vi "测量流程.vi"(11 "控制命令":T1(ring)) -> ()   [LabVIEW 2016, in "斯坦道总磷总氮.lvlib"]
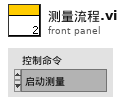
[diagram p1: front panel]
types:
  T1 = enum16{"启动测量", "标样核查", "零点核查", "跨度核查", "空白测试", "平行样测试", "加标回收", "空白校准", "标样校准", "初始化（清洗）", "停止测试", "仪器重启", "校时", "模式设置", "测量间隔设置"}
  T2 = typedef "斯坦道总磷总氮.lvlib/测试流程控件.ctl" = enum16{"初始化", "参数1启动", "参数1测试中", "参数1测试结束", "参数2启动", "参数2测试中", "参数2测试结束", "参数3启动", "参数3测试中", "参数3测试结束", "流程结束"}
  T3 = cluster{"时间标识":timestamp, "设备":string, "日志信息":string, "流程参数":string}
  T4 = cluster{"站号":u16, "量程切换":enum32{"H", "L", "AUTO"}, "控制命令":enum16{"启动测量", "标样核查", "零点核查", "跨度核查", "空白测试", "平行样测试", "加标回收", "空白校准", "标样校准", "初始化（清洗）", "停止测试", "仪器重启", "校时", "模式设置", "测量间隔设置"}, "模式设置":enum16{"待机", "连续模式", "周期模式", "定点模式", "受控模式", "手动模式"}, "测量间隔":u16}
  T5 = enum16{"空闲", "水样测试", "标样核查", "零点核查", "跨度核查", "空白测试", "平行样测试", "加标回收", "空白校准", "标样校准", "初始化（清洗）"}
  T6 = cluster{"系统时间":timestamp, "工作状态":enum16{"空闲", "水样测试", "标样核查", "零点核查", "跨度核查", "空白测试", "平行样测试", "加标回收", "空白校准", "标样校准", "初始化（清洗）"}, "测量模式":enum16{"待机", "连续模式", "周期模式", "定点模式", "受控模式", "手动模式"}, "告警代码":enum16{"无告警", "缺试剂告警", "缺水样告警", "缺蒸馏水告警", "缺标液告警", "仪表漏液告警", "标定异常告警", "超量程告警", "加热异常", "低试剂预警", "超上限告警", "超下限告警", "仪表内部其他异常", "滴定异常告警", "电极异常告警", "量程切换告警", "参数设置告警", "PH电极电位异常", "电导率电极异常", "浊度光度异常", "溶解氧电极异常", "溶解氧光强异常", "温度异常告警", "PH异常告警", "溶解氧异常告警", "电导率异常告警", "浊度异常告警", "叶绿素异常告警", "藻密度异常告警", "蓝绿藻异常告警", "ORP异常告警", "氨氮异常告警", "清洁刷异常告警", "SD卡异常告警", "蓝牙异常告警", "Wifi异常告警", "流程异常告警"}, "故障代码":enum16{"无故障", "电机故障", "温度故障", "通讯故障", "滴定故障"}, "日志代码":u16, "软件版本":u16, "F0":sgl, "F1":sgl, "F2":sgl, "F3":sgl, "T":sgl, "H":sgl, "id":u16, "flowid":u16, "量程":u16, "总磷控温温度1":sgl, "营养盐控温温度2":sgl, "ADC":sgl}
  T7 = cluster{"水样测试量程模式":enum16{"H", "L", "AUTO"}, "空白核查量程模式":enum16{"H", "L", "AUTO"}, "跨度核查量程模式":enum16{"H", "L", "AUTO"}}
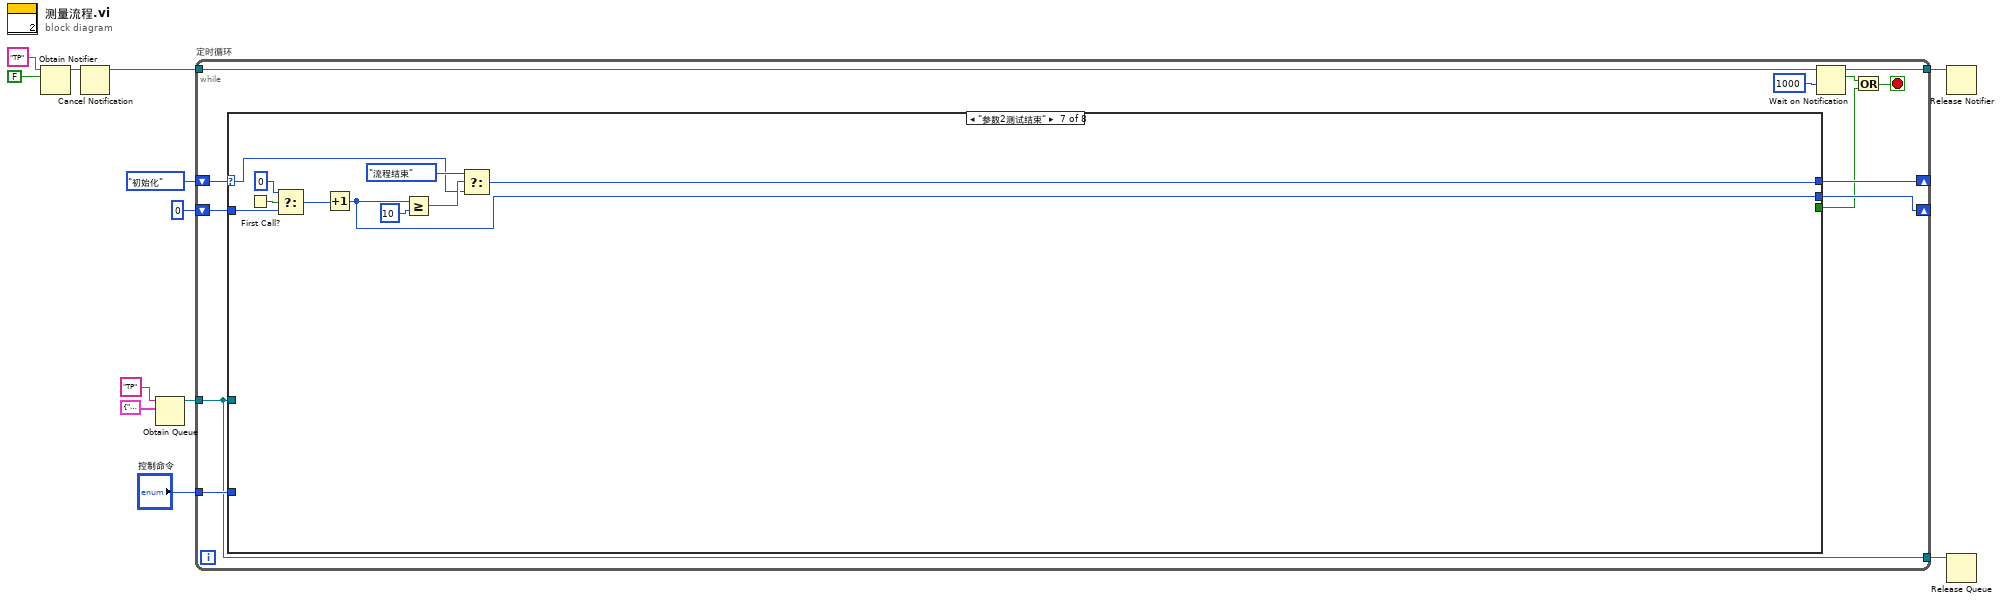
[diagram p0: block diagram]
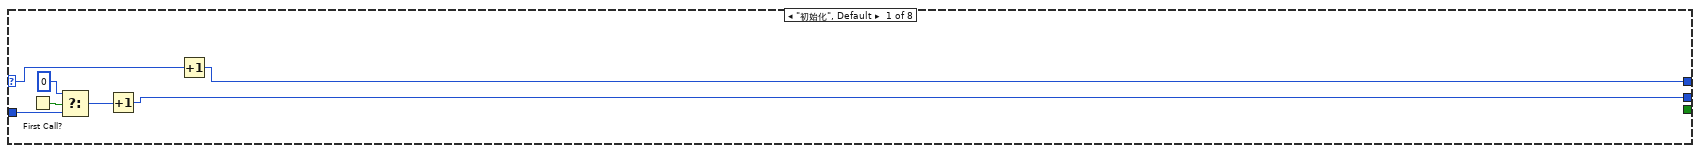
[diagram p2: hidden frame]
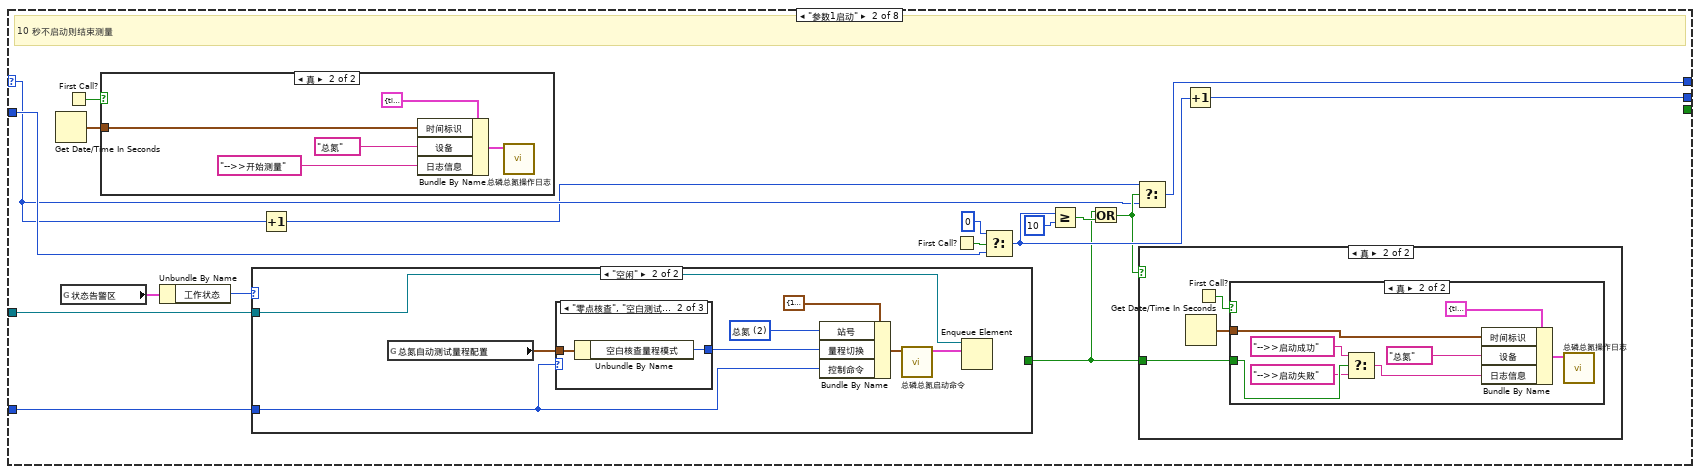
[diagram p3: hidden frame]
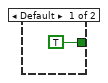
[diagram p7: hidden frame]
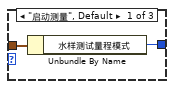
[diagram p8: hidden frame]
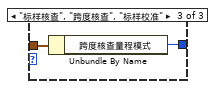
[diagram p9: hidden frame]
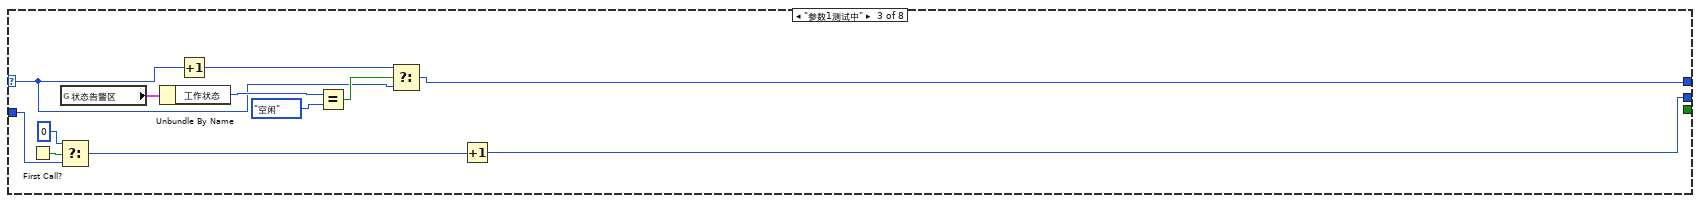
[diagram p10: hidden frame]
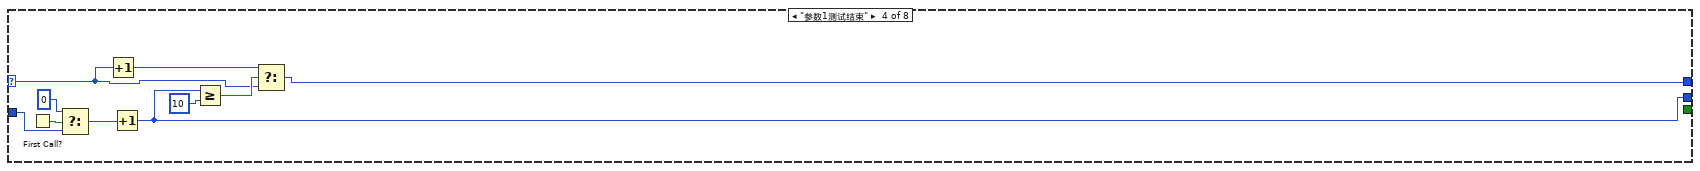
[diagram p11: hidden frame]
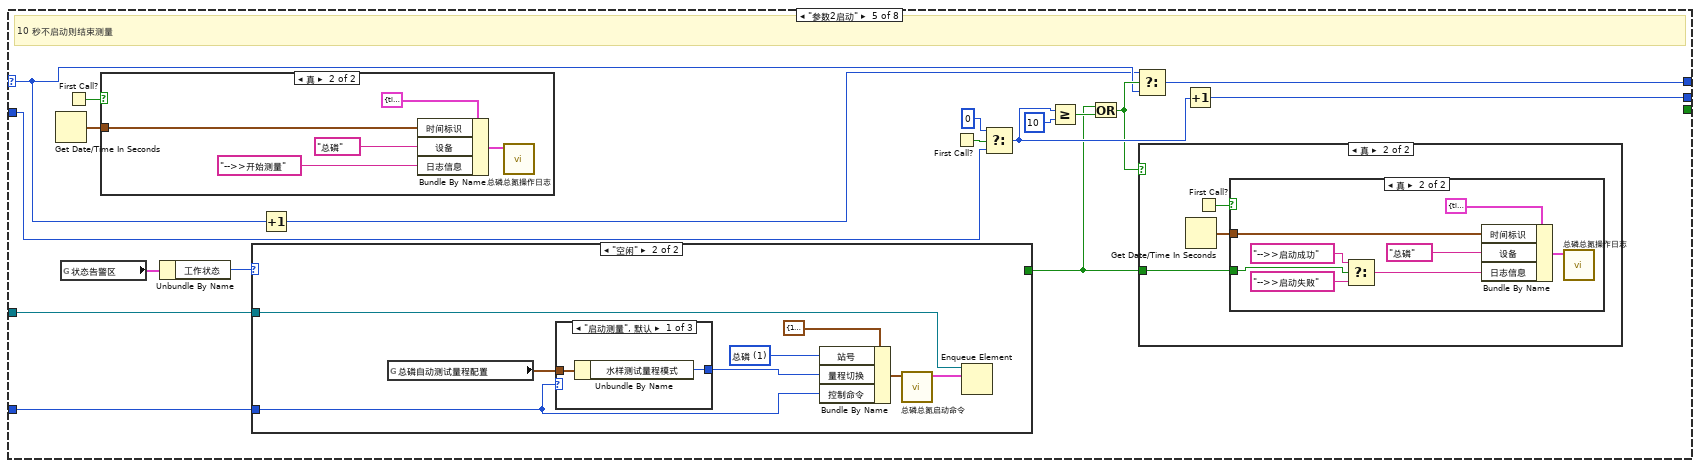
[diagram p12: hidden frame]
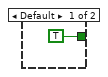
[diagram p16: hidden frame]
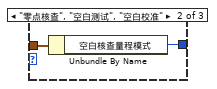
[diagram p17: hidden frame]
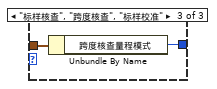
[diagram p18: hidden frame]
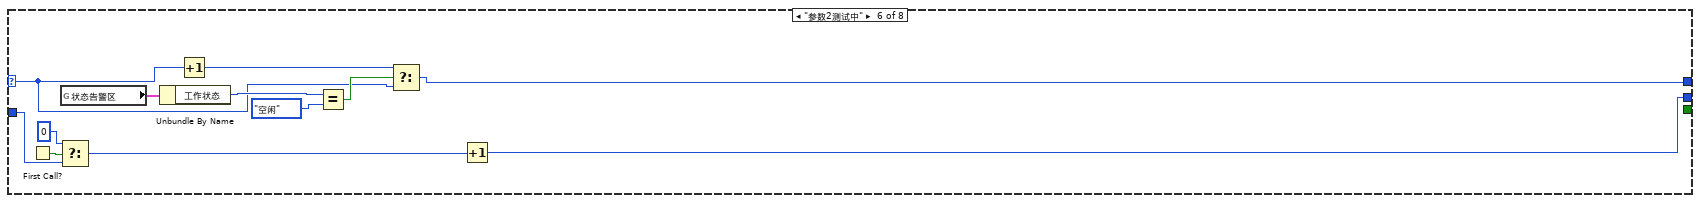
[diagram p19: hidden frame]
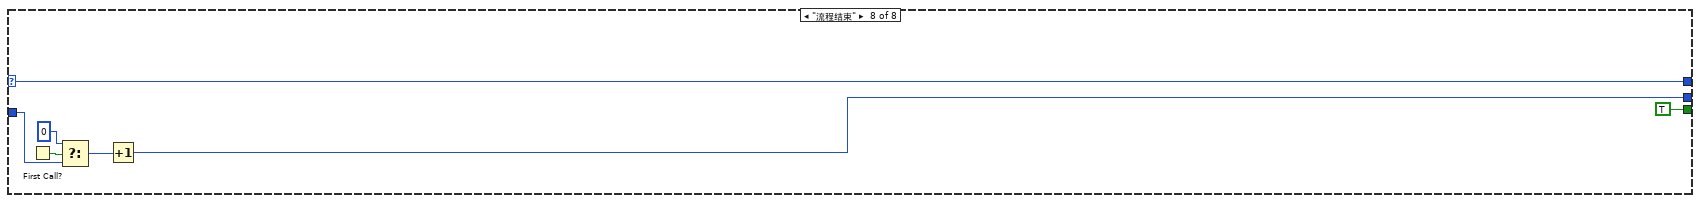
[diagram p20: hidden frame]
diagram:
  n1 = Obtain Notifier(name (unnamed)="TP" ("名称（未命名）"), notification data type=FALSE) -> (notifier out=w7:refnum<notifier>)  [unwired: 2 in, 2 out]
  n2 = Cancel Notification(0:w7) -> (8:w6:refnum<notifier>)  [unwired: 1 in, 2 out]
  n3 = Obtain Queue(name (unnamed)="TP" ("名称（未命名）"), element data type=cluster{"命令":string, "data":variant} {"命令"="", "data"=variant}) -> (queue out=w10:refnum<queue>)  [unwired: 3 in, 2 out]
  n4 = while "定时循环" {
    tunnel: w10 -> [w13]
    tunnel: w6 -> [w24]
    tunnel: "控制命令" -> [w19]
    shift-right: [w18] -> _
    shift-left: 测试流程控件."初始化" -> [w20]
    shift-right: [w16] -> _
    shift-left: 0 -> [w17]
    tunnel: [w14] -> w2
    tunnel: [w13] -> w3
    stop <- w21 stop-if-true
    n5 = case shown="\"参数2测试结束\"" w20 {
      selector: w20 -> [w31 w35 w83 w94 w106 w154 w165 w179]
      tunnel: w19 -> [_ w49 _ _ w120 _ _ _]
      tunnel: w13 -> [_ w48 _ _ w119 _ _ _]
      tunnel: [w30 w39 w84 w93 w110 w155 w164 w179] -> w18
      tunnel: w17 -> [w28 w43 w90 w100 w114 w161 w171 w175]
      tunnel: [w25 w42 w81 w98 w113 w152 w169 w174] -> w16
      tunnel: [_ _ _ _ _ _ _ TRUE] -> w15
      frame "初始化", Default {
        n6 = First Call?() -> (First Call?: T/F=w29:bool)
        n7 = Select(t=0, s=w29, f=w28) -> (s? t:f=w26:i32)
        n8 = Increment(x=w26) -> (x+1=w25:i32)
        n9 = Increment(x=w31) -> (x+1=w30:T2)
      }
      frame "参数1启动" {
        # "10 秒不启动则结束测量"
        n10 = Get Date/Time In Seconds() -> (seconds since 1Jan1904=w33:timestamp)
        n11 = global read "VAR总磷总氮全局变量.vi" "状态告警区"() -> (w47:T6)
        n12 = First Call?() -> (First Call?: T/F=w32:bool)
        n13 = case shown="真" w32 {
          tunnel: w33 -> [_ w53]
          frame False {
          }
          frame True {
            n14 = Bundle By Name(cluster=T3 {"时间标识"=timestamp(0 s since 1904-01-01), "设备"="", "日志信息"="", "流程参数"=""} ("data in"), "时间标识"=w53, "设备"="总氮" ("组合框"), "日志信息"="-->>开始测量") -> (w54:T3)
            n15 = call "总磷总氮操作日志.vi"("data in"=w54) -> ()  [unwired: 11 in]
          }
        }
        n16 = Unbundle By Name(w47) -> ("工作状态"=w46:T5)
        n17 = case shown="\"空闲\"" w46 {
          tunnel: w49 -> [_ w68]
          tunnel: w48 -> [_ w72]
          tunnel: [TRUE _] -> w36
          frame Default {
          }
          frame "空闲" {
            w71 = u16 2 items=["总磷"=1, "总氮"=2, "氨氮"=3, "COD"=22] ("站号")
            n18 = global read "总磷总氮断电保存全局变量.vi" "总氮自动测试量程配置"() -> (w67:T7)
            n19 = case shown="\"零点核查\", \"空白测试\", \"空白校准\"" w68 {
              tunnel: w67 -> [w76 w78 w80]
              tunnel: [w75 w77 w79] -> w74
              frame "启动测量", Default {
                n20 = Unbundle By Name(w76) -> ("水样测试量程模式"=w75:enum16{"H", "L", "AUTO"})
              }
              frame "零点核查", "空白测试", "空白校准" {
                n21 = Unbundle By Name(w78) -> ("空白核查量程模式"=w77:enum16{"H", "L", "AUTO"})
              }
              frame "标样核查", "跨度核查", "标样校准" {
                n22 = Unbundle By Name(w80) -> ("跨度核查量程模式"=w79:enum16{"H", "L", "AUTO"})
              }
            }
            n23 = Bundle By Name(cluster=T4 {"站号"=1, "量程切换"=enum."AUTO", "控制命令"=enum."启动测量", "模式设置"=enum."待机", "测量间隔"=0} ("参数"), "站号"=w71, "量程切换"=w74, "控制命令"=w68) -> (w69:T4)
            n24 = call "总磷总氮启动命令.vi"("参数"=w69) -> ("启动命令"=w73:cluster{"命令":string, "data":variant})  [unwired: 10 in]
            n25 = Enqueue Element(queue=w72, element=w73) -> ()  [unwired: 2 in, 3 out]
          }
        }
        n26 = Increment(x=w35) -> (x+1=w34:T2)
        n27 = First Call?() -> (First Call?: T/F=w45:bool)
        n28 = Select(t=0, s=w45, f=w43) -> (s? t:f=w41:i32)
        n29 = Greater Or Equal?(x=w41, y=10) -> (x >= y?=w38:bool)
        n30 = Or(x=w36, y=w38) -> (x .or. y?=w37:bool)
        n31 = Select(t=w34, s=w37, f=w35) -> (s? t:f=w39:T2)
        n32 = case shown="真" w37 {
          tunnel: w36 -> [_ w55]
          frame False {
          }
          frame True {
            n33 = Get Date/Time In Seconds() -> (seconds since 1Jan1904=w56:timestamp)
            n34 = First Call?() -> (First Call?: T/F=w57:bool)
            n35 = case shown="真" w57 {
              tunnel: w56 -> [_ w64]
              tunnel: w55 -> [_ w62]
              frame False {
              }
              frame True {
                n36 = Select(t="-->>启动成功" ("日志信息"), s=w62, f="-->>启动失败" ("日志信息")) -> (s? t:f=w59:string)
                n37 = Bundle By Name(cluster=T3 {"时间标识"=timestamp(0 s since 1904-01-01), "设备"="", "日志信息"="", "流程参数"=""} ("data in"), "时间标识"=w64, "设备"="总氮" ("组合框"), "日志信息"=w59) -> (w65:T3)
                n38 = call "总磷总氮操作日志.vi"("data in"=w65) -> ()  [unwired: 11 in]
              }
            }
          }
        }
        n39 = Increment(x=w41) -> (x+1=w42:i32)
      }
      frame "参数1测试中" {
        n40 = First Call?() -> (First Call?: T/F=w92:bool)
        n41 = Select(t=0, s=w92, f=w90) -> (s? t:f=w89:i32)
        n42 = global read "VAR总磷总氮全局变量.vi" "状态告警区"() -> (w88:T6)
        n43 = Unbundle By Name(w88) -> ("工作状态"=w87:T5)
        n44 = Increment(x=w83) -> (x+1=w82:T2)
        n45 = Equal?(x=w87, y=T5."空闲") -> (x = y?=w85:bool)
        n46 = Select(t=w82, s=w85, f=w83) -> (s? t:f=w84:T2)
        n47 = Increment(x=w89) -> (x+1=w81:i32)
      }
      frame "参数1测试结束" {
        n48 = First Call?() -> (First Call?: T/F=w102:bool)
        n49 = Select(t=0, s=w102, f=w100) -> (s? t:f=w99:i32)
        n50 = Increment(x=w94) -> (x+1=w95:T2)
        n51 = Increment(x=w99) -> (x+1=w98:i32)
        n52 = Greater Or Equal?(x=w98, y=10) -> (x >= y?=w96:bool)
        n53 = Select(t=w95, s=w96, f=w94) -> (s? t:f=w93:T2)
      }
      frame "参数2启动" {
        # "10 秒不启动则结束测量"
        n54 = Get Date/Time In Seconds() -> (seconds since 1Jan1904=w104:timestamp)
        n55 = global read "VAR总磷总氮全局变量.vi" "状态告警区"() -> (w118:T6)
        n56 = First Call?() -> (First Call?: T/F=w103:bool)
        n57 = case shown="真" w103 {
          tunnel: w104 -> [_ w124]
          frame False {
          }
          frame True {
            n58 = Bundle By Name(cluster=T3 {"时间标识"=timestamp(0 s since 1904-01-01), "设备"="", "日志信息"="", "流程参数"=""} ("data in"), "时间标识"=w124, "设备"="总磷" ("组合框"), "日志信息"="-->>开始测量") -> (w125:T3)
            n59 = call "总磷总氮操作日志.vi"("data in"=w125) -> ()  [unwired: 11 in]
          }
        }
        n60 = Unbundle By Name(w118) -> ("工作状态"=w117:T5)
        n61 = case shown="\"空闲\"" w117 {
          tunnel: w120 -> [_ w139]
          tunnel: w119 -> [_ w143]
          tunnel: [TRUE _] -> w107
          frame Default {
          }
          frame "空闲" {
            w142 = u16 1 items=["总磷"=1, "总氮"=2, "氨氮"=3, "COD"=22] ("站号")
            n62 = global read "总磷总氮断电保存全局变量.vi" "总磷自动测试量程配置"() -> (w138:T7)
            n63 = case shown="\"启动测量\", 默认" w139 {
              tunnel: w138 -> [w147 w149 w151]
              tunnel: [w146 w148 w150] -> w145
              frame "启动测量", Default {
                n64 = Unbundle By Name(w147) -> ("水样测试量程模式"=w146:enum16{"H", "L", "AUTO"})
              }
              frame "零点核查", "空白测试", "空白校准" {
                n65 = Unbundle By Name(w149) -> ("空白核查量程模式"=w148:enum16{"H", "L", "AUTO"})
              }
              frame "标样核查", "跨度核查", "标样校准" {
                n66 = Unbundle By Name(w151) -> ("跨度核查量程模式"=w150:enum16{"H", "L", "AUTO"})
              }
            }
            n67 = Bundle By Name(cluster=T4 {"站号"=1, "量程切换"=enum."AUTO", "控制命令"=enum."启动测量", "模式设置"=enum."待机", "测量间隔"=0} ("参数"), "站号"=w142, "量程切换"=w145, "控制命令"=w139) -> (w140:T4)
            n68 = call "总磷总氮启动命令.vi"("参数"=w140) -> ("启动命令"=w144:cluster{"命令":string, "data":variant})  [unwired: 10 in]
            n69 = Enqueue Element(queue=w143, element=w144) -> ()  [unwired: 2 in, 3 out]
          }
        }
        n70 = Increment(x=w106) -> (x+1=w105:T2)
        n71 = First Call?() -> (First Call?: T/F=w116:bool)
        n72 = Select(t=0, s=w116, f=w114) -> (s? t:f=w112:i32)
        n73 = Greater Or Equal?(x=w112, y=10) -> (x >= y?=w109:bool)
        n74 = Or(x=w107, y=w109) -> (x .or. y?=w108:bool)
        n75 = Select(t=w105, s=w108, f=w106) -> (s? t:f=w110:T2)
        n76 = case shown="真" w108 {
          tunnel: w107 -> [_ w126]
          frame False {
          }
          frame True {
            n77 = Get Date/Time In Seconds() -> (seconds since 1Jan1904=w127:timestamp)
            n78 = First Call?() -> (First Call?: T/F=w128:bool)
            n79 = case shown="真" w128 {
              tunnel: w127 -> [_ w135]
              tunnel: w126 -> [_ w133]
              frame False {
              }
              frame True {
                n80 = Select(t="-->>启动成功" ("日志信息"), s=w133, f="-->>启动失败" ("日志信息")) -> (s? t:f=w130:string)
                n81 = Bundle By Name(cluster=T3 {"时间标识"=timestamp(0 s since 1904-01-01), "设备"="", "日志信息"="", "流程参数"=""} ("data in"), "时间标识"=w135, "设备"="总磷" ("组合框"), "日志信息"=w130) -> (w136:T3)
                n82 = call "总磷总氮操作日志.vi"("data in"=w136) -> ()  [unwired: 11 in]
              }
            }
          }
        }
        n83 = Increment(x=w112) -> (x+1=w113:i32)
      }
      frame "参数2测试中" {
        n84 = First Call?() -> (First Call?: T/F=w163:bool)
        n85 = Select(t=0, s=w163, f=w161) -> (s? t:f=w160:i32)
        n86 = global read "VAR总磷总氮全局变量.vi" "状态告警区"() -> (w159:T6)
        n87 = Unbundle By Name(w159) -> ("工作状态"=w158:T5)
        n88 = Increment(x=w154) -> (x+1=w153:T2)
        n89 = Equal?(x=w158, y=T5."空闲") -> (x = y?=w156:bool)
        n90 = Select(t=w153, s=w156, f=w154) -> (s? t:f=w155:T2)
        n91 = Increment(x=w160) -> (x+1=w152:i32)
      }
      frame "参数2测试结束" {
        n92 = First Call?() -> (First Call?: T/F=w173:bool)
        n93 = Select(t=0, s=w173, f=w171) -> (s? t:f=w170:i32)
        n94 = Increment(x=w170) -> (x+1=w169:i32)
        n95 = Greater Or Equal?(x=w169, y=10) -> (x >= y?=w167:bool)
        n96 = Select(t=测试流程控件."流程结束", s=w167, f=w165) -> (s? t:f=w164:T2)
      }
      frame "流程结束" {
        n97 = First Call?() -> (First Call?: T/F=w178:bool)
        n98 = Select(t=0, s=w178, f=w175) -> (s? t:f=w176:i32)
        n99 = Increment(x=w176) -> (x+1=w174:i32)
      }
    }
    n100 = Wait on Notification(notifier=w24, timeout in ms (-1)=1000 ("超时毫秒(-1)")) -> (notifier out=w14:refnum<notifier>, notification=w22:bool)  [unwired: 2 in, 2 out]
    n101 = Or(x=w22, y=w15) -> (x .or. y?=w21:bool)
  }
  n102 = Release Notifier(notifier=w2) -> ()  [unwired: 2 in, 3 out]
  n103 = Release Queue(queue=w3) -> ()  [unwired: 2 in, 3 out]
